vi "format_CCSymbols_for_project.vi"(11 "CCSymbols":map{string, string}(c390)) -> (3 "CCSymbols for project":string)   [LabVIEW 2019]
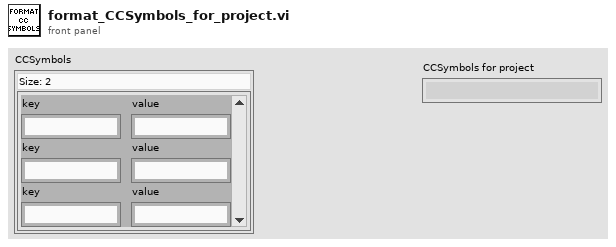
[diagram p1: front panel]
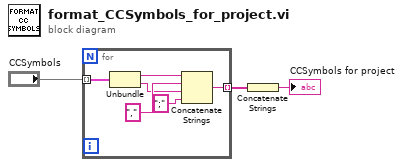
[diagram p0: block diagram]
diagram:
  n1 = for {
    tunnel: "CCSymbols" -> [w9] mode=indexing
    tunnel: [w4] -> w2 mode=indexing
    n2 = Unbundle(w9) -> ("key"=w8:string, "value"=w6:string)
    n3 = Concatenate Strings(w8, "," ("string"), w6, ";" ("string")) -> (w4:string)
  }
  n4 = Concatenate Strings(w2) -> (→"CCSymbols for project":string)
